vi "get_all_collections.vi"(0 "vector_qdrant in":refnum<class "vector_qdrant.lvclass">, 11 "error in (no error)":errorcluster) -> (4 "vector_qdrant out":refnum<class "vector_qdrant.lvclass">, 6 "collection":string[](array[string]), 15 "error out":errorcluster)   [LabVIEW 2020, in "vector_qdrant.lvclass"]
uses:
  vector_qdrant.lvclass
  vector_qdrant.lvclass/vector_qdrant.ctl
  <vilib>/httpClient/LabVIEWHTTPClient.lvlib
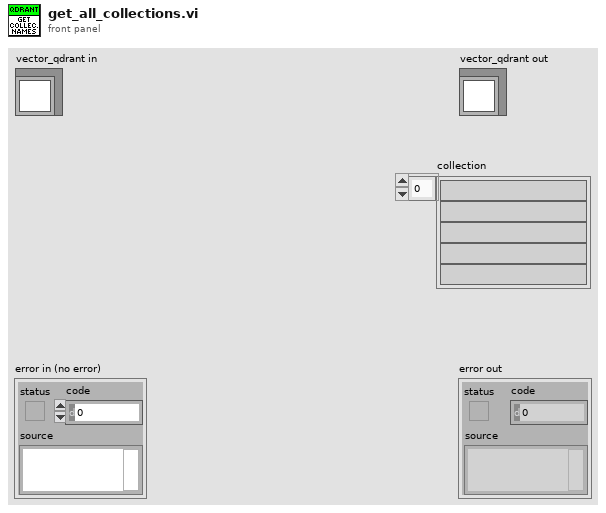
[diagram p1: front panel]
types:
  T1 = typedef "LabVIEWHTTPClient.lvlib/ClientHandle.ctl" = refnum<k1>
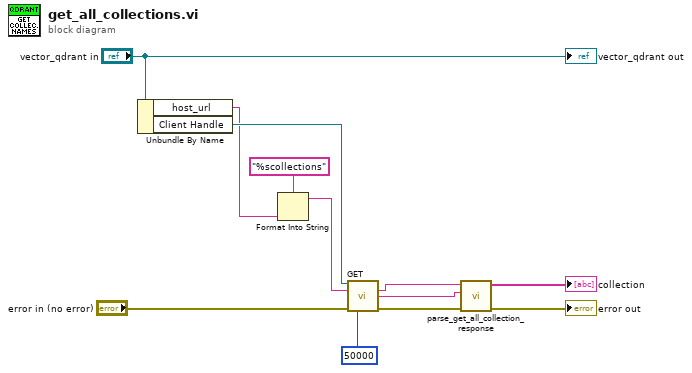
[diagram p0: block diagram]
diagram:
  n1 = Unbundle By Name("vector_qdrant in") -> ("host_url"=w8:string, "Client Handle"=w10:T1)
  n2 = Format Into String(format string="%scollections", w8) -> (resulting string=w7:string)  [unwired: 2 in, 1 out]
  n3 = call <vilib>:"GET.vi"("client handle"=w10, "url"=w7, "error in (no error)"="error in (no error)", "timeout (10000)"=50000) -> ("headers"=w3:string, "body"=w2:string, "error out"=w5:errorcluster)  [unwired: 8 in, 1 out]
  n4 = call "parse_get_all_collection_response.vi"("error in (no error)"=w5, "body"=w2, "headers"=w3) -> ("error out"=→"error out":errorcluster, "collection_list"=→"collection":string[])  [unwired: 7 in]
  "vector_qdrant out" <- "vector_qdrant in"
